vi "decryptVerify.vi"(0 "HGF_GPG":refnum<class "HGF_GPG.lvclass">, 1 "options file":path, 2 "keyringfile":path, 3 "Sec keyringfile":path, 4 "string in":string, 5 "error in (no error)":errorcluster, 6 "Trust DB":path, 7 "password":string) -> (8 "dup Trust DB":path, 10 "trusted":bool, 11 "success":bool=TRUE, 12 "Key-ID":string, 13 "data error":bool, 14 "dup HGF_GPG":refnum<class "HGF_GPG.lvclass">, 15 "dup options file":path, 16 "dup keyringfile":path, 17 "dup Sec keyringfile":path, 18 "String":string, 19 "error out":errorcluster)   [LabVIEW 2012, in "HGF_GPG.lvlib" / "HGF_GPG.lvclass"]
doc: "Decrypt and verify a string.\nIf the string is just crypted, it will only be encrypted, but no key id will be returned.\n\nIf no password is set, the private password will be used."
uses:
  HGF_GPG.lvclass
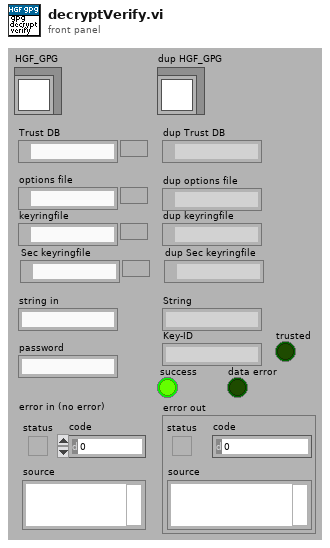
[diagram p1: front panel]
types:
  T1 = enum16{"open", "replace", "create", "open or create", "replace or create", "replace or create with confirmation"}
  T2 = enum16{"encrypt", "decrypt", "sign", "verify", "sign & encrypt", "verify & decrypt"}
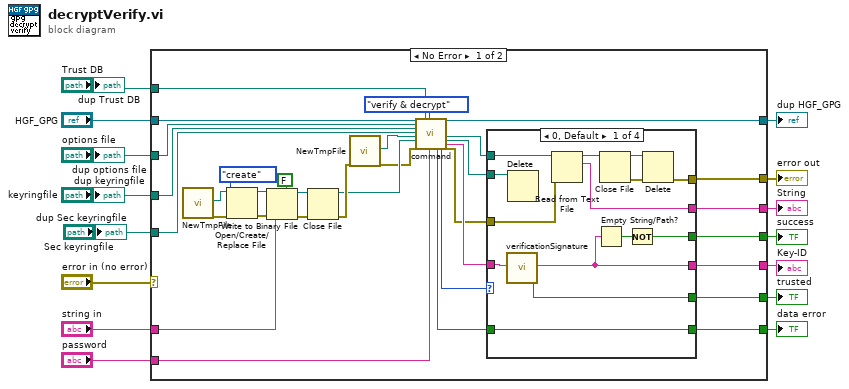
[diagram p0: block diagram]
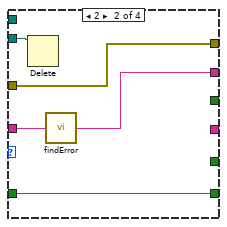
[diagram p2: hidden frame]
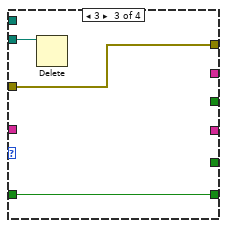
[diagram p3: hidden frame]
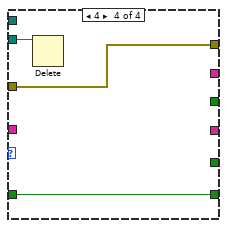
[diagram p4: hidden frame]
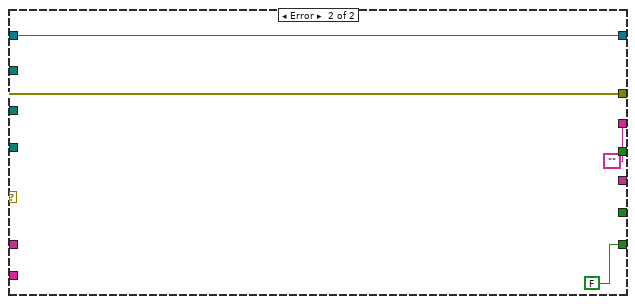
[diagram p5: hidden frame]
diagram:
  n1 = case shown="No Error" "error in (no error)" {
    selector: "error in (no error)" -> [_ w76]
    tunnel: [w45 w77] -> w13
    tunnel: "HGF_GPG" -> [w46 w77]
    tunnel: "password" -> [w26 _]
    tunnel: "string in" -> [w32 _]
    tunnel: [w40 ""] -> w10
    tunnel: [w39 w76] -> w9
    tunnel: [w34 _] -> w8
    tunnel: [w33 FALSE ("data error")] -> w7
    tunnel: [w31 _] -> w6
    tunnel: [w30 _] -> w5
    tunnel: "options file" -> [w28 _]
    tunnel: "keyringfile" -> [w27 _]
    tunnel: "Sec keyringfile" -> [w22 _]
    tunnel: "Trust DB" -> [w16 _]
    frame No Error {
      n2 = call "NewTmpFile.vi"() -> ("path"=w20:path, "error out"=w21:errorcluster)  [unwired: 1 in, 17 out]
      n3 = Open/Create/Replace File(file path (use dialog)=w20, error in=w21, operation (0:open)=T1."create") -> (refnum out=w36:refnum<file>, error out=w37:errorcluster)  [unwired: 4 out]
      n4 = Write to Binary File(file (use dialog)=w36, data=w32, error in=w37, 5:FALSE ("prepend array or string size? (T)")) -> (refnum out=w43:refnum<file>, error out=w44:errorcluster)  [unwired: 3 out]
      n5 = Close File(refnum=w43, error in=w44) -> (path=w19:path, error out=w48:errorcluster)
      n6 = call "NewTmpFile.vi"("error in (no error)"=w48) -> ("path"=w18:path, "error out"=w17:errorcluster)  [unwired: 17 out]
      n7 = call-dynamic "command.vi"("HGF_GPG"=w46, "options file"=w28, "keyringfile"=w27, "Sec keyringfile"=w22, "targetfile"=w18, "sourcefile"=w19, "error in (no error)"=w17, "Trust DB"=w16, "task"=T2."verify & decrypt", "password"=w26) -> ("data error"=w41:bool, "return code"=w25:i32, "dup HGF_GPG"=w45:refnum<class "HGF_GPG.lvclass">, "dup targetfile"=w23:path, "dup sourcefile"=w24:path, "standard error"=w47:string, "error out"=w42:errorcluster)  [unwired: 3 in, 8 out]
      n8 = case shown="0, Default" w25 {
        tunnel: w42 -> [w58 w67 w70 w73]
        tunnel: w41 -> [w57 w66 w69 w72]
        tunnel: [w52 w64 _ _] -> w40
        tunnel: [w59 w67 w70 w73] -> w39
        tunnel: [w50 _ _ _] -> w34
        tunnel: [w57 w66 w69 w72] -> w33
        tunnel: [w56 _ _ _] -> w31
        tunnel: [w49 _ _ _] -> w30
        tunnel: w47 -> [w55 w65 _ _]
        tunnel: w24 -> [w54 w63 w68 w71]
        tunnel: w23 -> [w53 _ _ _]
        frame 0, Default {
          n9 = call "verificationSignature.vi"("String"=w55) -> ("Key-ID"=w49:string, "trusted"=w56:bool)  [unwired: 17 out]
          n10 = Delete(path (use dialog)=w54) -> ()  [unwired: 1 in, 6 out]
          n11 = Read from Text File(file (use dialog)=w53, error in=w58) -> (refnum out=w62:refnum<file>, text=w52:string)  [unwired: 4 out]
          n12 = Empty String/Path?(string/path=w49) -> (empty?=w51:bool)
          n13 = Close File(refnum=w62) -> (path=w60:path, error out=w61:errorcluster)  [unwired: 1 in]
          n14 = Not(x=w51) -> (.not. x?=w50:bool)
          n15 = Delete(path (use dialog)=w60, error in=w61) -> (error out=w59:errorcluster)  [unwired: 5 out]
        }
        frame 2 {
          n16 = Delete(path (use dialog)=w63) -> ()  [unwired: 1 in, 6 out]
          n17 = call "findError.vi"("error string in"=w65) -> ("error out"=w64:string)
        }
        frame 3 {
          n18 = Delete(path (use dialog)=w68) -> ()  [unwired: 1 in, 6 out]
        }
        frame 4 {
          n19 = Delete(path (use dialog)=w71) -> ()  [unwired: 1 in, 6 out]
        }
      }
    }
    frame Error {
    }
  }
  "dup HGF_GPG" <- w13
  "String" <- w10
  "error out" <- w9
  "success" <- w8
  "data error" <- w7
  "trusted" <- w6
  "Key-ID" <- w5
  "dup options file" <- "options file"
  "dup keyringfile" <- "keyringfile"
  "dup Sec keyringfile" <- "Sec keyringfile"
  "dup Trust DB" <- "Trust DB"
